vi "subHamamatsu_GetMaxFrameRate.vi"(7 "ROI in":T1={"Bin"=2, "ROI"={"x offset"=256, "y offset"=256, "x width"=512, "y width"=512}} caption="ROI" {"ROI"."x offset" min=1 max=512 step=1; "ROI"."y offset" min=1 max=512 step=1; "ROI"."x width" min=1 max=512 step=1; "ROI"."y width" min=1 max=512 step=1; "Bin" items=["1x1"=1, "2x2"=2, "4x4"=4]}, 8 "error in":errorcluster, 11 "Handle in":u32) -> (0 "error out":errorcluster, 3 "Handle out":u32, 5 "max frame rate (Hz)":dbl=1425.0)   [LabVIEW 2015]
panel:
  # "Calculate theoretical maximum camera rate"
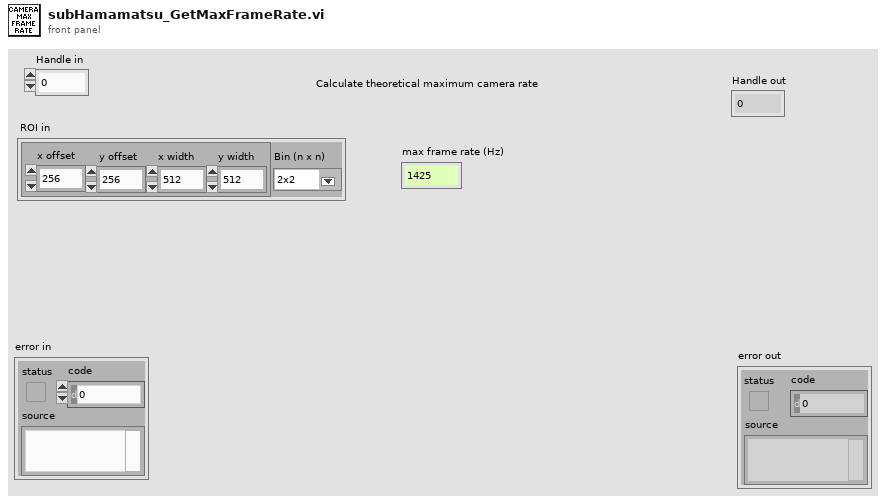
[diagram p1: front panel]
types:
  T1 = cluster{"Bin":u16, "ROI":cluster{"x offset":i32, "y offset":i32, "x width":i32, "y width":i32}}
  T2 = cluster{"x offset":i32, "y offset":i32, "x width":i32, "y width":i32}
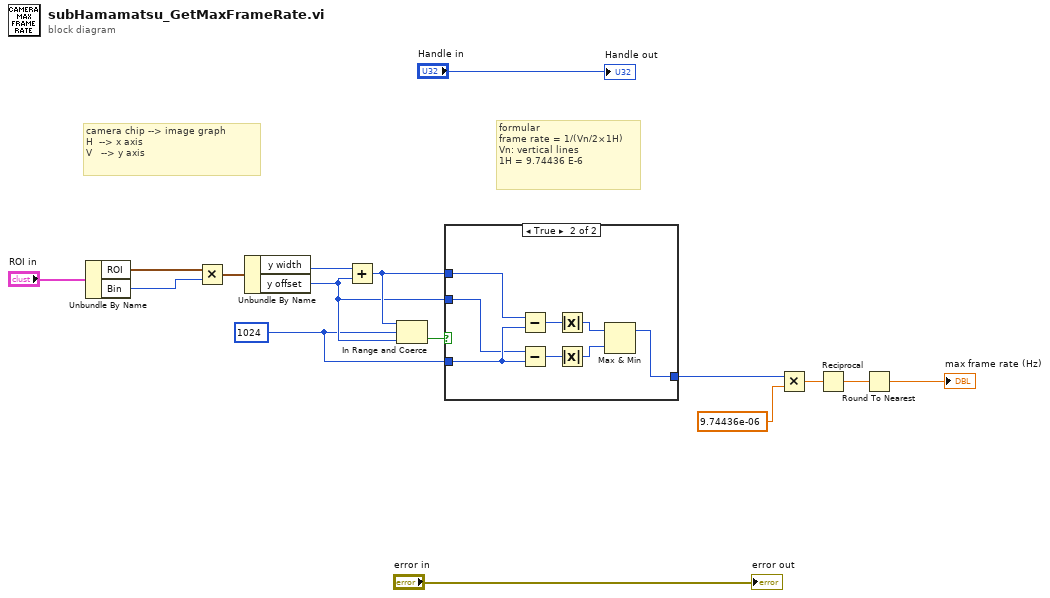
[diagram p0: block diagram]
diagram:
  w6 = 1024 ("Binned pixels")
  # "camera chip --> image graph\nH  --> x axis\nV   --> y axis"
  # "formular\nframe rate = 1/(Vn/2×1H)\nVn: vertical lines\n1H = 9.74436 E-6"
  n1 = Unbundle By Name("ROI in") -> ("ROI"=w5:T2, "Bin"=w4:u16)
  n2 = Multiply(x=w5, y=w4) -> (x*y=w7:T2)
  n3 = Unbundle By Name(w7) -> ("y width"=w15:i32, "y offset"=w13:i32)
  n4 = Add(x=w15, y=w13) -> (x+y=w14:i32)
  n5 = In Range and Coerce(upper limit=w14, x=w6, lower limit=w13) -> (In Range?=w16:bool)  [unwired: 1 out]
  n6 = case shown="True" w16 {
    tunnel: w13 -> [_ w18]
    tunnel: [w17 w21] -> w11
    tunnel: w6 -> [_ w20]
    tunnel: w14 -> [w17 w19]
    frame False {
    }
    frame True {
      n7 = Subtract(x=w19, y=w20) -> (x-y=w22:i32)
      n8 = Subtract(x=w18, y=w20) -> (x-y=w23:i32)
      n9 = Absolute Value(x=w22) -> (abs(x)=w24:i32)
      n10 = Absolute Value(x=w23) -> (abs(x)=w25:i32)
      n11 = Max & Min(x=w24, y=w25) -> (max(x,y)=w21:i32)  [unwired: 1 out]
    }
  }
  n12 = Multiply(x=w11, y=9.74436e-06) -> (x*y=w12:dbl)
  n13 = Reciprocal(x=w12) -> (1/x=w9:dbl)
  n14 = Round To Nearest(number=w9) -> (nearest integer value=→"max frame rate (Hz)":dbl)
  "error out" <- "error in"
  "Handle out" <- "Handle in"
